vi "NanotecSMCPDDriver.get position.vi"(0 "VISA resource name":refnum<visa-resource-name>, 1 "contollerID":i32=-1, 5 "error in (no error)":errorcluster) -> (14 "VISA resource name out":refnum<visa-resource-name>, 15 "contollerID out":i32=-1, 17 "actPosition [usteps]":i32, 19 "error out":errorcluster)   [LabVIEW 2014, in "NanotecSMCPDDriver.lvlib"]
doc: "Gets the actual position."
uses:
  NanotecSMCPDDriver.lvlib
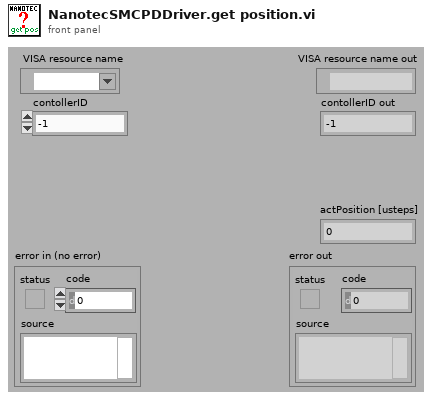
[diagram p1: front panel]
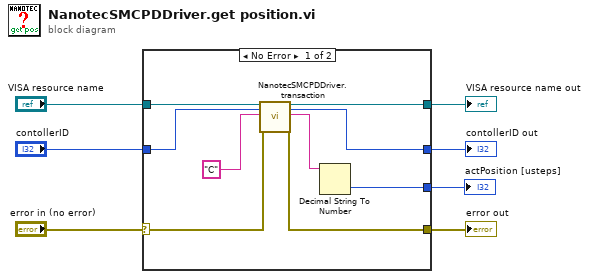
[diagram p0: block diagram]
diagram:
  n1 = case shown="No Error" "error in (no error)" {
    selector: "error in (no error)" -> [w9 w17]
    tunnel: [w12 w19] -> w7
    tunnel: [w10 w17] -> w6
    tunnel: "VISA resource name" -> [w16 w19]
    tunnel: "contollerID" -> [w14 w18]
    tunnel: [w13 w18] -> w3
    tunnel: [w8 _] -> w1
    frame No Error {
      n2 = call "NanotecSMCPDDriver.transaction.vi"("VISAresource"=w16, "contollerID"=w14, "commandString"="C", "error in (no error)"=w9) -> ("VISAresource out"=w12:refnum<visa-resource-name>, "contollerID out"=w13:i32, "response"=w11:string, "error out"=w10:errorcluster)  [unwired: 10 in, 2 out]
      n3 = Decimal String To Number(string=w11) -> (number=w8:i32)  [unwired: 2 in, 1 out]
    }
    frame Error {
    }
  }
  "VISA resource name out" <- w7
  "error out" <- w6
  "contollerID out" <- w3
  "actPosition [usteps]" <- w1
